vi "Log fill data.vi"(6 "component":string, 8 "time":timestamp[](array[timestamp]) format="%<%x %.3X>T", 9 "temp":dbl[](array[numeric]), 10 "press":dbl[](array[numeric]), 11 "tdms file":refnum<k34>) -> (3 "tdms file out":refnum<k34>)   [LabVIEW 2018]
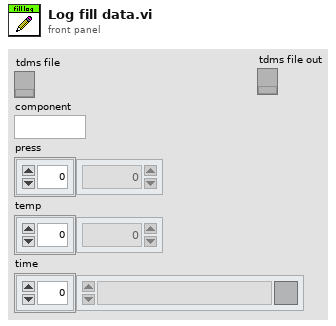
[diagram p1: front panel]
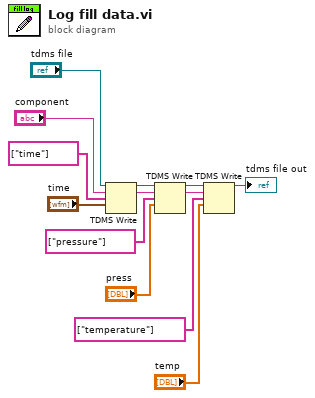
[diagram p0: block diagram]
diagram:
  n1 = TDMS Write(0:"tdms file", 5:"component", 7:string[] ["time"] ("channel name(s) in (Untitled)"), 9:"time") -> (4:w12:refnum<k34>, 6:w9:string)  [unwired: 2 in, 2 out]
  n2 = TDMS Write(0:w12, 5:w9, 7:string[] ["pressure"] ("channel name(s) in (Untitled)"), 9:"press") -> (4:w11:refnum<k34>, 6:w8:string)  [unwired: 2 in, 2 out]
  n3 = TDMS Write(0:w11, 5:w8, 7:string[] ["temperature"] ("channel name(s) in (Untitled)"), 9:"temp") -> (4:→"tdms file out":refnum<k34>)  [unwired: 2 in, 3 out]
